vi "Gill_chksum.vi"(0 "Address":string, 1 "Gill string":string) -> (3 "Stripped string":string, 4 "Error Notes":string)   [LabVIEW 2010]
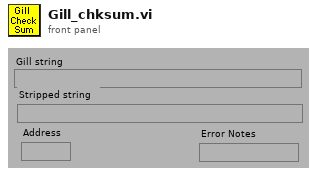
[diagram p1: front panel]
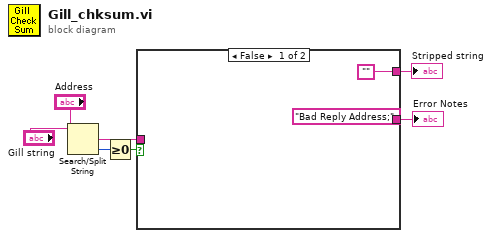
[diagram p0: block diagram]
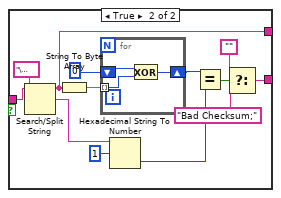
[diagram p2: hidden frame]
diagram:
  n1 = Search/Split String(string="Gill string", search string/char (-)="Address") -> (match + rest of string=w5:string, offset of match=w4:i32)  [unwired: 2 out]
  n2 = Greater Or Equal To 0?(x=w4) -> (x >= 0?=w3:bool)
  n3 = case shown="False" w3 {
    tunnel: w5 -> [_ w21]
    tunnel: ["Bad Reply Address;" w14] -> w2
    tunnel: ["" w10] -> w1
    frame False {
    }
    frame True {
      n4 = Search/Split String(string=w21, search string/char (-)="\u0003" ("search char (-)")) -> (substring before match=w10:string, match + rest of string=w22:string)  [unwired: 2 out]
      n5 = String To Byte Array(string=w10) -> (unsigned byte array=w16:u8[])
      n6 = for {
        tunnel: w16 -> [w25] mode=indexing
        shift-right: [w24] -> w17
        shift-left: u8 0 -> [w23]
        n7 = Exclusive Or(1:w25, 2:w23) -> (0:w24:u8)
      }
      n8 = Hexadecimal String To Number(string=w22, offset=1) -> (number=w18:u32)  [unwired: 2 out]
      n9 = Equal?(x=w17, y=w18) -> (x = y?=w13:bool)
      n10 = Select(t="", s=w13, f="Bad Checksum;") -> (s? t:f=w14:string)
    }
  }
  "Error Notes" <- w2
  "Stripped string" <- w1
